vi "Teleop Shooter Control.vi"(8 "Manipulator D-Pad":T2, 9 "Manipulator Buttons":T3, 10 "Driver Buttons":T3, 11 "Manipulator Axes":T1) -> ()   [LabVIEW 2015]
uses:
  Common Code/Gamepads/Button Cluster.ctl
  Common Code/Gamepads/D-Pad.ctl
  Common Code/Gamepads/Axes Cluster.ctl
  Common Code/Shooter Commands.ctl
  Common Code/Change Detect Boolean.vi
  Robot Global Data.vi
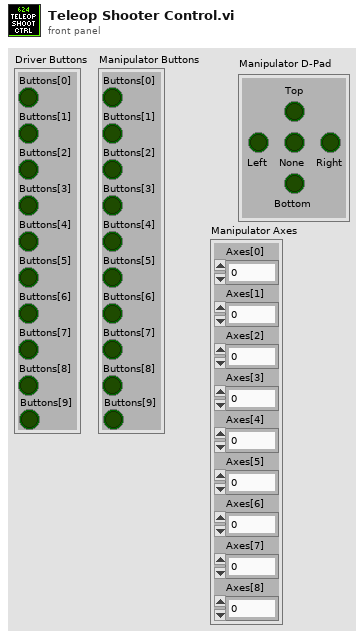
[diagram p1: front panel]
types:
  T1 = typedef "Axes Cluster.ctl" = cluster{"Axes[0]":dbl, "Axes[1]":dbl, "Axes[2]":dbl, "Axes[3]":dbl, "Axes[4]":dbl, "Axes[5]":dbl, "Axes[6]":dbl, "Axes[7]":dbl, "Axes[8]":dbl}
  T2 = typedef "D-Pad.ctl" = cluster{"Top":bool, "Bottom":bool, "None":bool, "Right":bool, "Left":bool}
  T3 = typedef "Button Cluster.ctl" = cluster{"Buttons[0]":bool, "Buttons[1]":bool, "Buttons[2]":bool, "Buttons[3]":bool, "Buttons[4]":bool, "Buttons[5]":bool, "Buttons[6]":bool, "Buttons[7]":bool, "Buttons[8]":bool, "Buttons[9]":bool}
  T4 = typedef "Shoot Modes Enum.ctl" = enum16{"Manual", "Safe", "Auto"}
  T5 = typedef "Shooter Commands.ctl" = enum16{"Idle", "Prime Shooter", "Shoot"}
  T6 = typedef "Shot Type.ctl" = enum16{"Batter Shot", "Corner Shot", "Cleat Shot", "Vision Shot", "Deep Middle Shot"}
  T7 = typedef "Dashboard Control Data.ctl" = cluster{"Shooter Presets":T8, "Encoder Control":T10, "Steer PID output":cluster{"output high":dbl, "output low":dbl}, " Steer PID gains":cluster{"proportional gain (Kc)":dbl, "integral time (Ti, min)":dbl, "derivative time (Td, min)":dbl}, "Drivetrain Settings":T11, "Vision Packet":T12, "Dashboard Drivetrain Command":T13, "Info/Command Cluster":T15, "Ball Vision Packet":T16, "Intake Presets":T18, "Intake Encoder Control":T20, "Climb Presets":T21, "Goal Output Range":cluster{"output high":dbl, "output low":dbl}, "Enabled Systems":T22, "Auton Presets":T23, "Pressure M":dbl, "Pressure B":dbl, "Vision Timeout":dbl, "Auto-Shift":T24}
  T8 = typedef "Shooter Presets.ctl" = cluster{"Batter Shot":T9, "Deep Middle":T9, "Manual Shot":T9, "Left Ticks Per Rotation":dbl, "Right Ticks Per Rotation":dbl, "Low Bar Shot":T9, "Shooter RPM Tolerance":dbl, "Trigger Power":dbl, "Fire from Load Delay":i32, "Max Angle":dbl, "Min Angle":dbl, "Angle PID gains":cluster{"P":dbl, "I":dbl, "D":dbl}, "Angle Output":cluster{"output high":dbl, "output low":dbl}, "Shooter Angle Tolerance":dbl, "Vision Shoot x^2":dbl, "Vision Shoot x":dbl, "Feed Forward Max Accel":dbl, "Feed Forward Kv":dbl, "Backwards Trigger":dbl, "Shot Finish Delay (ms)":dbl, "Angle Max Current":dbl, "Angle Current Trip Time":dbl, "Intake Angle":dbl, "Vision Shoot c":dbl, "Reset?":bool, "Button Release Delay":dbl, "Angle Pot x":dbl, "Angle Pot c":dbl, "Ignore Angle?":bool, "Max RPM":dbl, "Safty Frist Angle":dbl, "Intake Danger Height":dbl, "Angle Pot B":i32, "Angle Pot M":dbl, "FF Finish RPM":dbl, "RPM PID Right":cluster{"P":dbl, "I":dbl, "D":dbl, "FF":dbl}, "RPM PID Left":cluster{"P":dbl, "I":dbl, "D":dbl, "FF":dbl}, "Backwards RPM":dbl, "Vision RPM":dbl, "Run Wheels Backward Delay":u32, "Cleat Shot":T9}
  T9 = typedef "Shot Presets.ctl" = cluster{"L":dbl, "R":dbl, "A":dbl}
  T10 = typedef "Encoder Control.ctl" = cluster{"Right Tick Constant":dbl, "Left Tick Constant":dbl, "Reset?":bool, "Y Dist":cluster{"PID gains":cluster{"proportional gain (Kc)":dbl, "integral time (Ti, min)":dbl, "derivative time (Td, min)":dbl}}, "Y Stop Thresh":dbl, "Y Stop Speed":dbl}
  T11 = typedef "Drivetrain Settings.ctl" = cluster{"Gyro Tolerance":dbl, "Throttle Ramp (ms)":dbl, "Kv":dbl, "Ka":dbl, "Feed Forward P":dbl, "Feed Forward D":dbl, "Goal Vision PID gains":cluster{"proportional gain (Kc)":dbl, "integral time (Ti, min)":dbl, "derivative time (Td, min)":dbl}, "Goal Detection Window":dbl, "Creep Rate":dbl, "Vision Throttle Threshold":dbl, "Min Turn Output":dbl, "Left Batter Angle":dbl, "Right Batter Angle":dbl}
  T12 = typedef "Goal Vision Packet.ctl" = cluster{"Distance":dbl, "Center X":dbl, "Center Y":dbl, "Found Target?":bool, "Robot Center":dbl, "Angle":dbl}
  T13 = typedef "Dashboard Drivetrain Command.ctl" = cluster{"Drivetrain Vision":T14}
  T14 = typedef "Drivetrain Vision.ctl" = cluster{"Goal Window":dbl, "Ball Window":dbl}
  T15 = typedef "Ball Tracking Command Cluster.ctl" = cluster{"Distance to Ball":dbl, "Desired Angle":dbl, "Command":enum16{"Turn to Ball", "Turn to Angle", "Get Distance"}, "Pixels from Center":dbl}
  T16 = typedef "Ball Vision Packet.ctl" = cluster{"Ball Detected?":bool, "Distance to Ball":dbl, "Desired Angle":dbl, "Pixels from Center":dbl, "Tracking mode":T17}
  T17 = typedef "Tracking Mode.ctl" = enum16{"Turn to Ball", "Turn to Angle"}
  T18 = typedef "Intake Presets.ctl" = cluster{"Intake Speed":dbl, "Outake Speed":dbl, "Low Height":dbl, "Half Height":dbl, "High Idle Height":dbl, "Angle Speed":dbl, "Angle Tolerance":dbl, "Encoder Scale":dbl, "Load Height":dbl, "Output Range":T19, "Rotation Power Max/Min":dbl, "MaxCurrent":dbl, "Intake Trip Time":dbl, "Idle Height":dbl, "Max Height":dbl, "Reset Encoders?":bool, "PID gains":cluster{"proportional gain (Kc)":dbl, "integral time (Ti, min)":dbl, "derivative time (Td, min)":dbl}, "Intake Stop Delay":u32, "Settle Time":dbl, "Settle Wait Time":dbl, "Pull Up Delay":dbl}
  T19 = typedef "Drivetrain Output Range.ctl" = cluster{"output high":dbl, "output low":dbl}
  T20 = typedef "IntakeEcoderControl.ctl" = cluster{"Arm Tick Constant":dbl, "Reset?":bool, "Y Dist":cluster{"PID gains":cluster{"proportional gain (Kc)":dbl, "integral time (Ti, min)":dbl, "derivative time (Td, min)":dbl}}, "Y Stop Thresh":dbl, "Y Stop Speed":dbl}
  T21 = typedef "Climb Presets.ctl" = cluster{"Pull Power":dbl, "Extend Power":dbl}
  T22 = typedef "Enabled Systems.ctl" = cluster{"Shoot":bool, "Intake":bool, "DT":bool, "Gyro":bool, "100ms":bool, "US":bool}
  T23 = typedef "Autonomous Presets.ctl" = cluster{"Pitch Limit":dbl, "Roll Limit":dbl, "Start Position":dbl, "Cross Position":dbl}
  T24 = typedef "Auto Shift Cluster.ctl" = cluster{"Delay":dbl, "Avg Speed L/R":dbl, "Speed Thresh":dbl, "Upshift Accel":dbl, "Upshift Throttle":dbl, "Upshift Throttle Accel":dbl, "Downshift Throttle":dbl, "Downshift Throttle Accel":dbl}
  T25 = typedef "Manual Shoot.ctl" = cluster{"Spin Wheels":bool, "Fire":bool, "Angle":dbl, "Angle Power":dbl, "Use Manual Angle":bool, "Override RPM":bool, "Left RPM":dbl, "Right RPM":dbl, "Secure Ball?":bool}
  T26 = typedef "Shooter Command Cluster.ctl" = cluster{"Command":T5, "Mode":T4, "Shot Type":T6, "Override Trigger Sensor":bool, "Override Angle?":bool, "Hide From Death":bool}
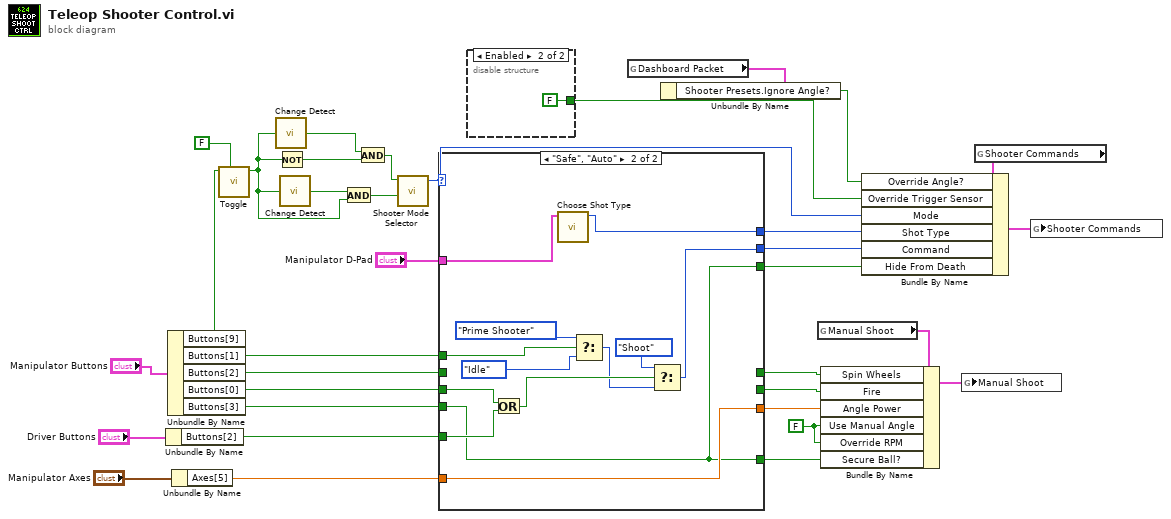
[diagram p0: block diagram]
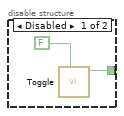
[diagram p2: hidden frame]
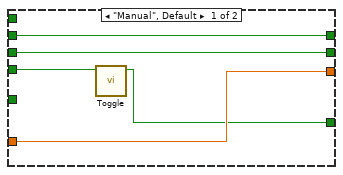
[diagram p3: hidden frame]
diagram:
  w16 = FALSE ("Use Manual Angle")
  n1 = Unbundle By Name("Driver Buttons") -> ("Buttons[2]"=w20:bool)
  n2 = Unbundle By Name("Manipulator Buttons") -> ("Buttons[9]"=w3:bool, "Buttons[1]"=w32:bool, "Buttons[2]"=w29:bool, "Buttons[0]"=w22:bool, "Buttons[3]"=w15:bool)
  n3 = Unbundle By Name("Manipulator Axes") -> ("Axes[5]"=w11:dbl)
  n4 = call "Toggle.vi"("Initial Value"=FALSE, "In"=w3) -> ("Toggled"=w4:bool)  [unwired: 9 in]
  n5 = call-poly "Change Detect.vi"("In"=w4) -> ("Changed?"=w8:bool)
  n6 = Not(x=w4) -> (.not. x?=w6:bool)
  n7 = call-poly "Change Detect.vi"("In"=w4) -> ("Changed?"=w5:bool)
  n8 = And(x=w5, y=w4) -> (x .and. y?=w2:bool)
  n9 = And(x=w8, y=w6) -> (x .and. y?=w1:bool)
  n10 = call "Shooter Mode Selector.vi"("Set To Manual?"=w2, "Set To Auto?"=w1) -> ("Mode"=w17:T4)  [unwired: 9 in]
  n11 = case shown="\"Safe\", \"Auto\"" w17 {
    tunnel: w32 -> [_ w49]
    tunnel: [_ w42] -> w31
    tunnel: w29 -> [w39 _]
    tunnel: [w39 _] -> w27
    tunnel: [w37 _] -> w25
    tunnel: "Manipulator D-Pad" -> [_ w51]
    tunnel: [_ w50] -> w23
    tunnel: w22 -> [w37 w47]
    tunnel: w20 -> [_ w46]
    tunnel: [w38 w44] -> w18
    tunnel: w11 -> [w38 w44]
    tunnel: w15 -> [w36 w40]
    tunnel: [w35 w40] -> w14
    tunnel: [_ w40] -> w9
    frame "Manual", Default {
      n12 = call "Toggle.vi"("In"=w36) -> ("Toggled"=w35:bool)  [unwired: 10 in]
    }
    frame "Safe", "Auto" {
      n13 = Or(x=w47, y=w46) -> (x .or. y?=w45:bool)
      n14 = call "Choose Shot Type.vi"("Manipulator D-Pad"=w51) -> ("Shot Type"=w50:T6)  [unwired: 10 in]
      n15 = Select(t=Shooter_Commands."Prime Shooter" ("Command"), s=w49, f=Shooter_Commands."Idle" ("Command")) -> (s? t:f=w41:T5)
      n16 = Select(t=Shooter_Commands."Shoot", s=w45, f=w41) -> (s? t:f=w42:T5)
    }
  }
  n17 = disable-structure shown="Enabled" {
    disable-tunnel: [w54 FALSE ("Toggled")] -> w10
    frame Disabled {
      n18 = call "Toggle.vi"("Initial Value"=FALSE) -> ("Toggled"=w54:bool)  [unwired: 10 in]
    }
    frame Enabled {
    }
  }
  n19 = global read "Robot Global Data.vi" "Dashboard Packet"() -> (w13:T7)
  n20 = Unbundle By Name(w13) -> ("Shooter Presets.Ignore Angle?"=w12:bool)
  n21 = global read "Robot Global Data.vi" "Manual Shoot"() -> (w28:T25)
  n22 = Bundle By Name(cluster=w28, "Spin Wheels"=w27, "Fire"=w25, "Angle Power"=w18, "Use Manual Angle"=w16, "Override RPM"=w16, "Secure Ball?"=w14) -> (w26:T25)
  n23 = global write "Robot Global Data.vi" "Manual Shoot"(w26) -> ()
  n24 = global read "Robot Global Data.vi" "Shooter Commands"() -> (w30:T26)
  n25 = Bundle By Name(cluster=w30, "Override Angle?"=w12, "Override Trigger Sensor"=w10, "Mode"=w17, "Shot Type"=w23, "Command"=w31, "Hide From Death"=w9) -> (w33:T26)
  n26 = global write "Robot Global Data.vi" "Shooter Commands"(w33) -> ()
